vi "sema4.vi"() -> ()   [LabVIEW 2013]
panel:
  out "C":bool
  out "B":bool
  out "A":bool
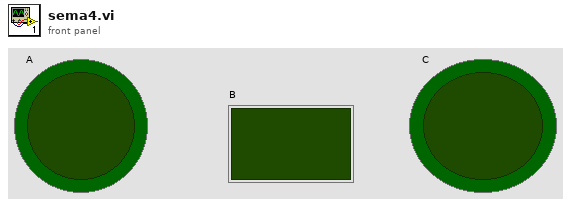
[diagram p1: front panel]
types:
  T1 = typedef "Semaphore RefNum" = refnum<k1>
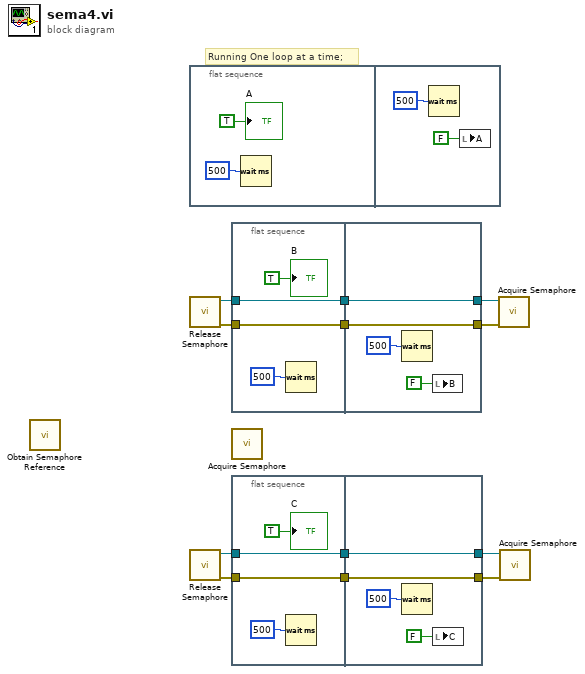
[diagram p0: block diagram]
diagram:
  # "Running One loop at a time;"
  n1 = call <vilib>:"Obtain Semaphore Reference.vi"() -> ()  [unwired: 5 in, 3 out]
  n2 = flat-sequence {
    frame #0 {
      n3 = Wait (ms)(milliseconds to wait=u32 500) -> ()  [unwired: 1 out]
      "A" <- TRUE ("A")
    }
    frame #1 {
      n4 = Wait (ms)(milliseconds to wait=u32 500) -> ()  [unwired: 1 out]
      n5 = local write "A"(FALSE ("A")) -> ()
    }
  }
  n6 = call <vilib>:"Release Semaphore.vi"() -> ("error out"=w8:errorcluster, "semaphore out"=w11:T1)  [unwired: 6 in]
  n7 = call <vilib>:"Release Semaphore.vi"() -> ("error out"=w2:errorcluster, "semaphore out"=w5:T1)  [unwired: 6 in]
  n8 = flat-sequence {
    tunnel: [w18] -> w12
    tunnel: w11 -> [w18]
    tunnel: [w17] -> w9
    tunnel: w8 -> [w17]
    tunnel: w12 -> [w22]
    tunnel: [w22] -> w10
    tunnel: w9 -> [w21]
    tunnel: [w21] -> w7
    frame #0 {
      n9 = Wait (ms)(milliseconds to wait=u32 500) -> ()  [unwired: 1 out]
      "B" <- TRUE ("B")
    }
    frame #1 {
      n10 = Wait (ms)(milliseconds to wait=u32 500) -> ()  [unwired: 1 out]
      n11 = local write "B"(FALSE ("B")) -> ()
    }
  }
  n12 = call <vilib>:"Acquire Semaphore.vi"() -> ()  [unwired: 5 in, 3 out]
  n13 = flat-sequence {
    tunnel: [w26] -> w6
    tunnel: w5 -> [w26]
    tunnel: [w25] -> w3
    tunnel: w2 -> [w25]
    tunnel: w6 -> [w30]
    tunnel: [w30] -> w4
    tunnel: w3 -> [w29]
    tunnel: [w29] -> w1
    frame #0 {
      n14 = Wait (ms)(milliseconds to wait=u32 500) -> ()  [unwired: 1 out]
      "C" <- TRUE ("C")
    }
    frame #1 {
      n15 = Wait (ms)(milliseconds to wait=u32 500) -> ()  [unwired: 1 out]
      n16 = local write "C"(FALSE ("C")) -> ()
    }
  }
  n17 = call <vilib>:"Acquire Semaphore.vi"("error in (no error)"=w7, "semaphore"=w10) -> ()  [unwired: 3 in, 3 out]
  n18 = call <vilib>:"Acquire Semaphore.vi"("error in (no error)"=w1, "semaphore"=w4) -> ()  [unwired: 3 in, 3 out]
